vi "GoToKick.vi"(1 "goleiro?":bool, 2 "Impulso ini.\npass state":bool=TRUE, 3 "balls":T4[](array[typedef]), 4 "Robot in in":T5={"id"=0, "function"=enum."Attacker", "x"=0.0, "y"=0.0, "orientation"=0.0, "v_tangent"=0.0, "v_normal"=0.0, "v_ang"=0.0, "kick_x"=0.0, "kick_z"=0.0, "dribble"=FALSE, "Timestamp"=timestamp(0 s since 1904-01-01), "estimatives"={"est_v_tangent"=0.0, "est_v_normal"=0.0, "est_vx"=0.0, "est_vy"=0.0, "Pos Robot Est"=[]}, "dest_x_kick"=0.0, "dest_y_kick"=0.0, "Gap Coord"=[], "States"=enum."Pass", "Path "=[], "Path  Smooth"=[], "Dest"=[]}, 5 "atacando contra?":bool, 6 "Field Size in":T3, 7 "Target":dbl[](array[numeric]), 8 "Defender":bool, 9 "D ball - robot":dbl, 10 "AI Parameters":T2={"GotoKick"={"Dist do cone a frente"=150.0, "attacker farback"=1500.0, "Perto"=300.0, "min dist to kick"=150.0, "kick eps"=0.05, "Time to transition"=0.0}, "Attacker"={"CC chute"=0.09, "CC passe"=0.045, "Kick Force"=100.0, "ball-robot Kick"=200.0, "ball-robot Pass"=0.3, "drible\nAttk"=FALSE}, "Defender"={"D max"=1700.0, "Vel p/ robô av"=1000.0, "Kick Force"=100.0, "D atk-def"=0.0, "D farback"=0.0, "drible\ndef"=FALSE, "drible\ngoalie"=FALSE}, "Timeout"={"Field/v in x"=6.0, "Dist Robots"=300, "Dist up in y"=300}, "Pose Striker"={"dist"=200.0, "Numeric"=-4.0, "dist 2"=200.0, "drible\nstriker"=FALSE}, "Dist Stop"=300.0, "D ball out"=200, "D central gap "=150.0, "T pass"=0.0, "Force ++"=0.0, "range kick"=0.0, "Chute alto"=TRUE, "Marcador novo"=TRUE, "drible"=FALSE, "D drible"=300.0, "Versão Striker"=enum."3", "Defesa"=enum."ManMark", "Marcador"=enum."Marcar Segundo mais perigoso", "Receptor passe"=enum."2nd Striker", "Área"=enum."Quadrada", "Decisão\nsimples?"=FALSE} {"D drible" format="%#_13g"; "D central gap" format="%#_13g"; "Dist Stop" format="%#_13g"; "Pose Striker"."Numeric" format="%#_13g"; "Defender"."Kick Force" format="%#_13g"; "Defender"."Vel p/ robô av" format="%#_13g"; "Attacker"."ball-robot Kick" format="%#_13g"; "Attacker"."Kick Force" format="%#_13g"; "Attacker"."CC passe" format="%#_13g"; "Attacker"."CC chute" format="%#_13g"; "GotoKick"."min dist to kick" format="%#_13g"; "GotoKick"."Perto" format="%#_13g"; "GotoKick"."attacker farback" format="%#_13g"; "GotoKick"."Dist do cone a frente" format="%#_13g"}, 11 "Cone de chute":dbl=0.09 format="%#_13g", 13 "Passe":bool, 16 "Personalidade":T1, 18 "Kick Force":dbl=5.0 format="%#_13g", 19 "IA State Input in":T10) -> (0 "Current States":T7, 12 "Next State":T7, 14 "Robot out":T5={"id"=0, "function"=enum."Attacker", "x"=0.0, "y"=0.0, "orientation"=0.0, "v_tangent"=0.0, "v_normal"=0.0, "v_ang"=0.0, "kick_x"=0.0, "kick_z"=0.0, "dribble"=FALSE, "Timestamp"=timestamp(0 s since 1904-01-01), "estimatives"={"est_v_tangent"=0.0, "est_v_normal"=0.0, "est_vx"=0.0, "est_vy"=0.0, "Pos Robot Est"=[]}, "dest_x_kick"=0.0, "dest_y_kick"=0.0, "Gap Coord"=[], "States"=enum."Pass", "Path "=[], "Path  Smooth"=[], "Dest"=[]}, 17 "kick error":dbl)   [LabVIEW 2018]
uses:
  Core/AI Input.ctl
  Core/AI Robot.ctl
  Functions Enum.ctl
  AttackerStates.ctl
  Path Planning/RRT/PathDests.ctl
  Path Planning/RRT/PathDest.ctl
  Core/AI Ball.ctl
  Core/Field Size.ctl
  Core/AI Judge.ctl
  Command Enum.ctl
  Util/Events/Events.ctl
  AI Parameters.ctl
  PersonalityEnum.ctl
  <vilib>/Analysis/_algsub.llb/Real Vector Norm.vi
  <vilib>/Analysis/baseanly.llb/Real Dot Product.vi
  <vilib>/Analysis/coordinate.llb/2D Cartesian Coordinate Rotation (Scalar).vi
  <vilib>/Analysis/NI_AALPro.lvlib
  <vilib>/Analysis/NI_AALBase.lvlib
panel:
  out "Elapsed Time (s)":dbl
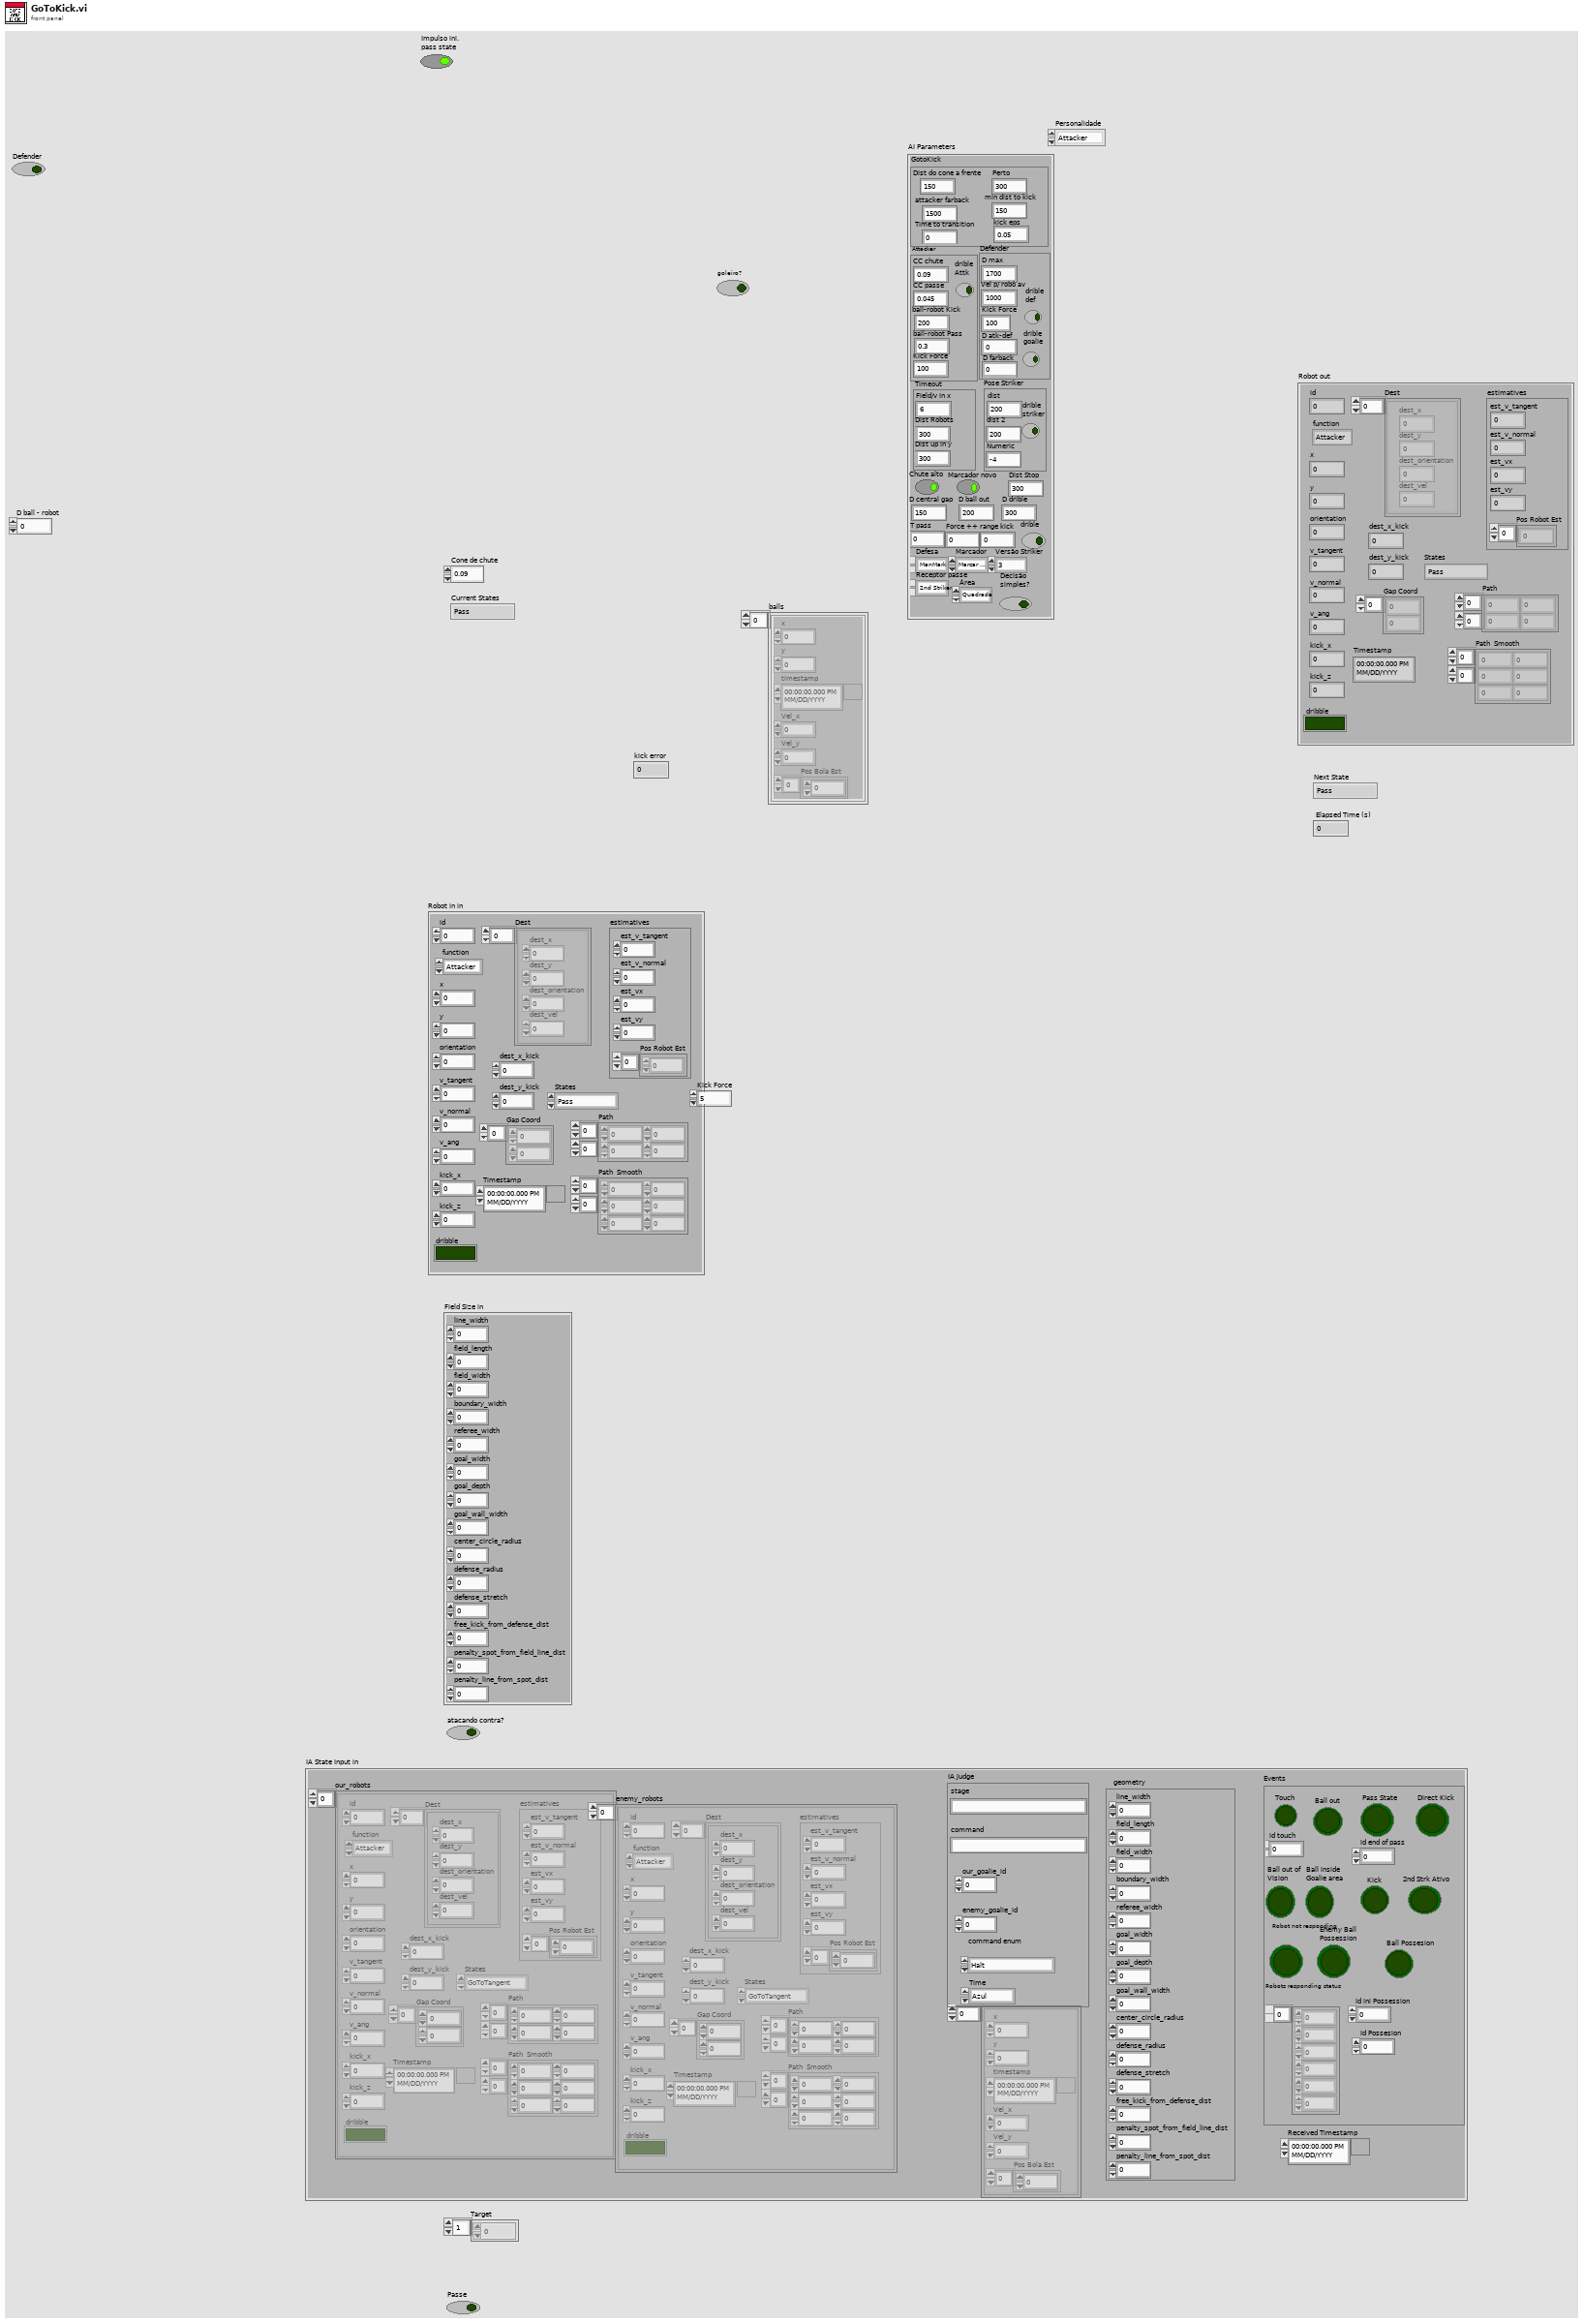
[diagram p1: front panel]
types:
  T1 = typedef "PersonalityEnum.ctl" = enum16{"Attacker", "Striker", "Defender", "Goalie"}
  T2 = typedef "AI Parameters.ctl" = cluster{"GotoKick":cluster{"Dist do cone a frente":dbl, "attacker farback":dbl, "Perto":dbl, "min dist to kick":dbl, "kick eps":dbl, "Time to transition":dbl}, "Attacker":cluster{"CC chute":dbl, "CC passe":dbl, "Kick Force":dbl, "ball-robot Kick":dbl, "ball-robot Pass":dbl, "drible\nAttk":bool}, "Defender":cluster{"D max":dbl, "Vel p/ robô av":dbl, "Kick Force":dbl, "D atk-def":dbl, "D farback":dbl, "drible\ndef":bool, "drible\ngoalie":bool}, "Timeout":cluster{"Field/v in x":dbl, "Dist Robots":u32, "Dist up in y":u32}, "Pose Striker":cluster{"dist":dbl, "Numeric":dbl, "dist 2":dbl, "drible\nstriker":bool}, "Dist Stop":dbl, "D ball out":i32, "D central gap ":dbl, "T pass":dbl, "Force ++":dbl, "range kick":dbl, "Chute alto":bool, "Marcador novo":bool, "drible":bool, "D drible":dbl, "Versão Striker":enum16{"Auto", "3", "2", "1"}, "Defesa":enum16{"ManMark", "Barreira"}, "Marcador":enum16{"Marcar Segundo mais perigoso", "Marcar o mais perigoso"}, "Receptor passe":enum16{"Auto", "2nd Striker", "Striker"}, "Área":enum16{"Quadrada", "Circular"}, "Decisão\nsimples?":bool}
  T3 = typedef "Field Size.ctl" = cluster{"line_width":u32, "field_length":u32, "field_width":u32, "boundary_width":u32, "referee_width":u32, "goal_width":u32, "goal_depth":u32, "goal_wall_width":u32, "center_circle_radius":u32, "defense_radius":u32, "defense_stretch":u32, "free_kick_from_defense_dist":u32, "penalty_spot_from_field_line_dist":u32, "penalty_line_from_spot_dist":u32}
  T4 = typedef "AI Ball.ctl" = cluster{"x":dbl, "y":dbl, "timestamp":timestamp, "Vel_x":dbl, "Vel_y":dbl, "Pos Bola Est":dbl[]}
  T5 = typedef "AI Robot.ctl" = cluster{"id":u32, "function":T6, "x":dbl, "y":dbl, "orientation":dbl, "v_tangent":dbl, "v_normal":dbl, "v_ang":dbl, "kick_x":dbl, "kick_z":dbl, "dribble":bool, "Timestamp":timestamp, "estimatives":cluster{"est_v_tangent":dbl, "est_v_normal":dbl, "est_vx":dbl, "est_vy":dbl, "Pos Robot Est":dbl[]}, "dest_x_kick":dbl, "dest_y_kick":dbl, "Gap Coord":dbl[], "States":T7, "Path ":dbl[][], "Path  Smooth":dbl[][], "Dest":T8}
  T6 = typedef "Functions Enum.ctl" = enum16{"2nd Striker", "Attacker", "Goalie", "Defender", "Striker", "Goto 0", "Dummy", "Kicker", "ZigZag 0", "ZigZag 1", "ZigZag 2", "ZigZag 3", "ZigZag 4", "ZigZag 5", "ZigZag 6", "ZigZag 7", "ZigZag 8", ""}
  T7 = typedef "AttackerStates.ctl" = enum16{"Pass", "GoToTangent", "BallGetting", "GoToKick", ""}
  T8 = typedef "PathDests.ctl" = T9[]
  T9 = typedef "PathDest.ctl" = cluster{"dest_x":dbl, "dest_y":dbl, "dest_orientation":dbl, "dest_vel":dbl}
  T10 = typedef "AI Input.ctl" = cluster{"our_robots":T5[], "enemy_robots":T5[], "balls":T4[], "geometry":T3, "IA Judge":T11, "Received Timestamp":timestamp, "Events":T13}
  T11 = typedef "AI Judge.ctl" = cluster{"stage":string, "command":string, "our_goalie_id":dbl, "enemy_goalie_id":dbl, "command enum":T12, "Time":enum16{"Azul", "Amarelo"}}
  T12 = typedef "Command Enum.ctl" = enum16{"Halt", "Stop", "Force Start", "PKA Normal Start", "Prepare Kickoff Ally", "PKE Normal Start", "Prepare Kickoff Enemy", "Prepare Penalty Ally", "PPA Normal Start", "Prepare Penalty Enemy", "PPE Normal Start", "Direct Free Enemy", "Direct Free Ally", "Indirect Free Enemy", "Indirect Free Ally", "Timeout Enemy", "Timeout Ally", "Goal Enemy", "Goal Ally", "Ball Placement Enemy", "Ball Placement Ally", "Normal Half Time", "Extra Time Break", "Extra Half Time", "None", "Post Game"}
  T13 = typedef "Events.ctl" = cluster{"Touch":bool, "Ball out":bool, "id touch":dbl, "Ball out of \nVision":bool, "Ball inside \nGoalie area":bool, "Robot not responding":bool, "Robots responding status":dbl[], "Enemy Ball \nPossession":bool, "Pass State":bool, "id end of pass":dbl, "Kick":bool, "Id ini Possession":dbl, "Ball Possesion":bool, "Id Possesion":dbl, "Direct Kick":bool, "2nd Strk Ativo":bool}
  T14 = cluster{"Dist do cone a frente":dbl, "attacker farback":dbl, "Perto":dbl, "min dist to kick":dbl, "kick eps":dbl, "Time to transition":dbl}
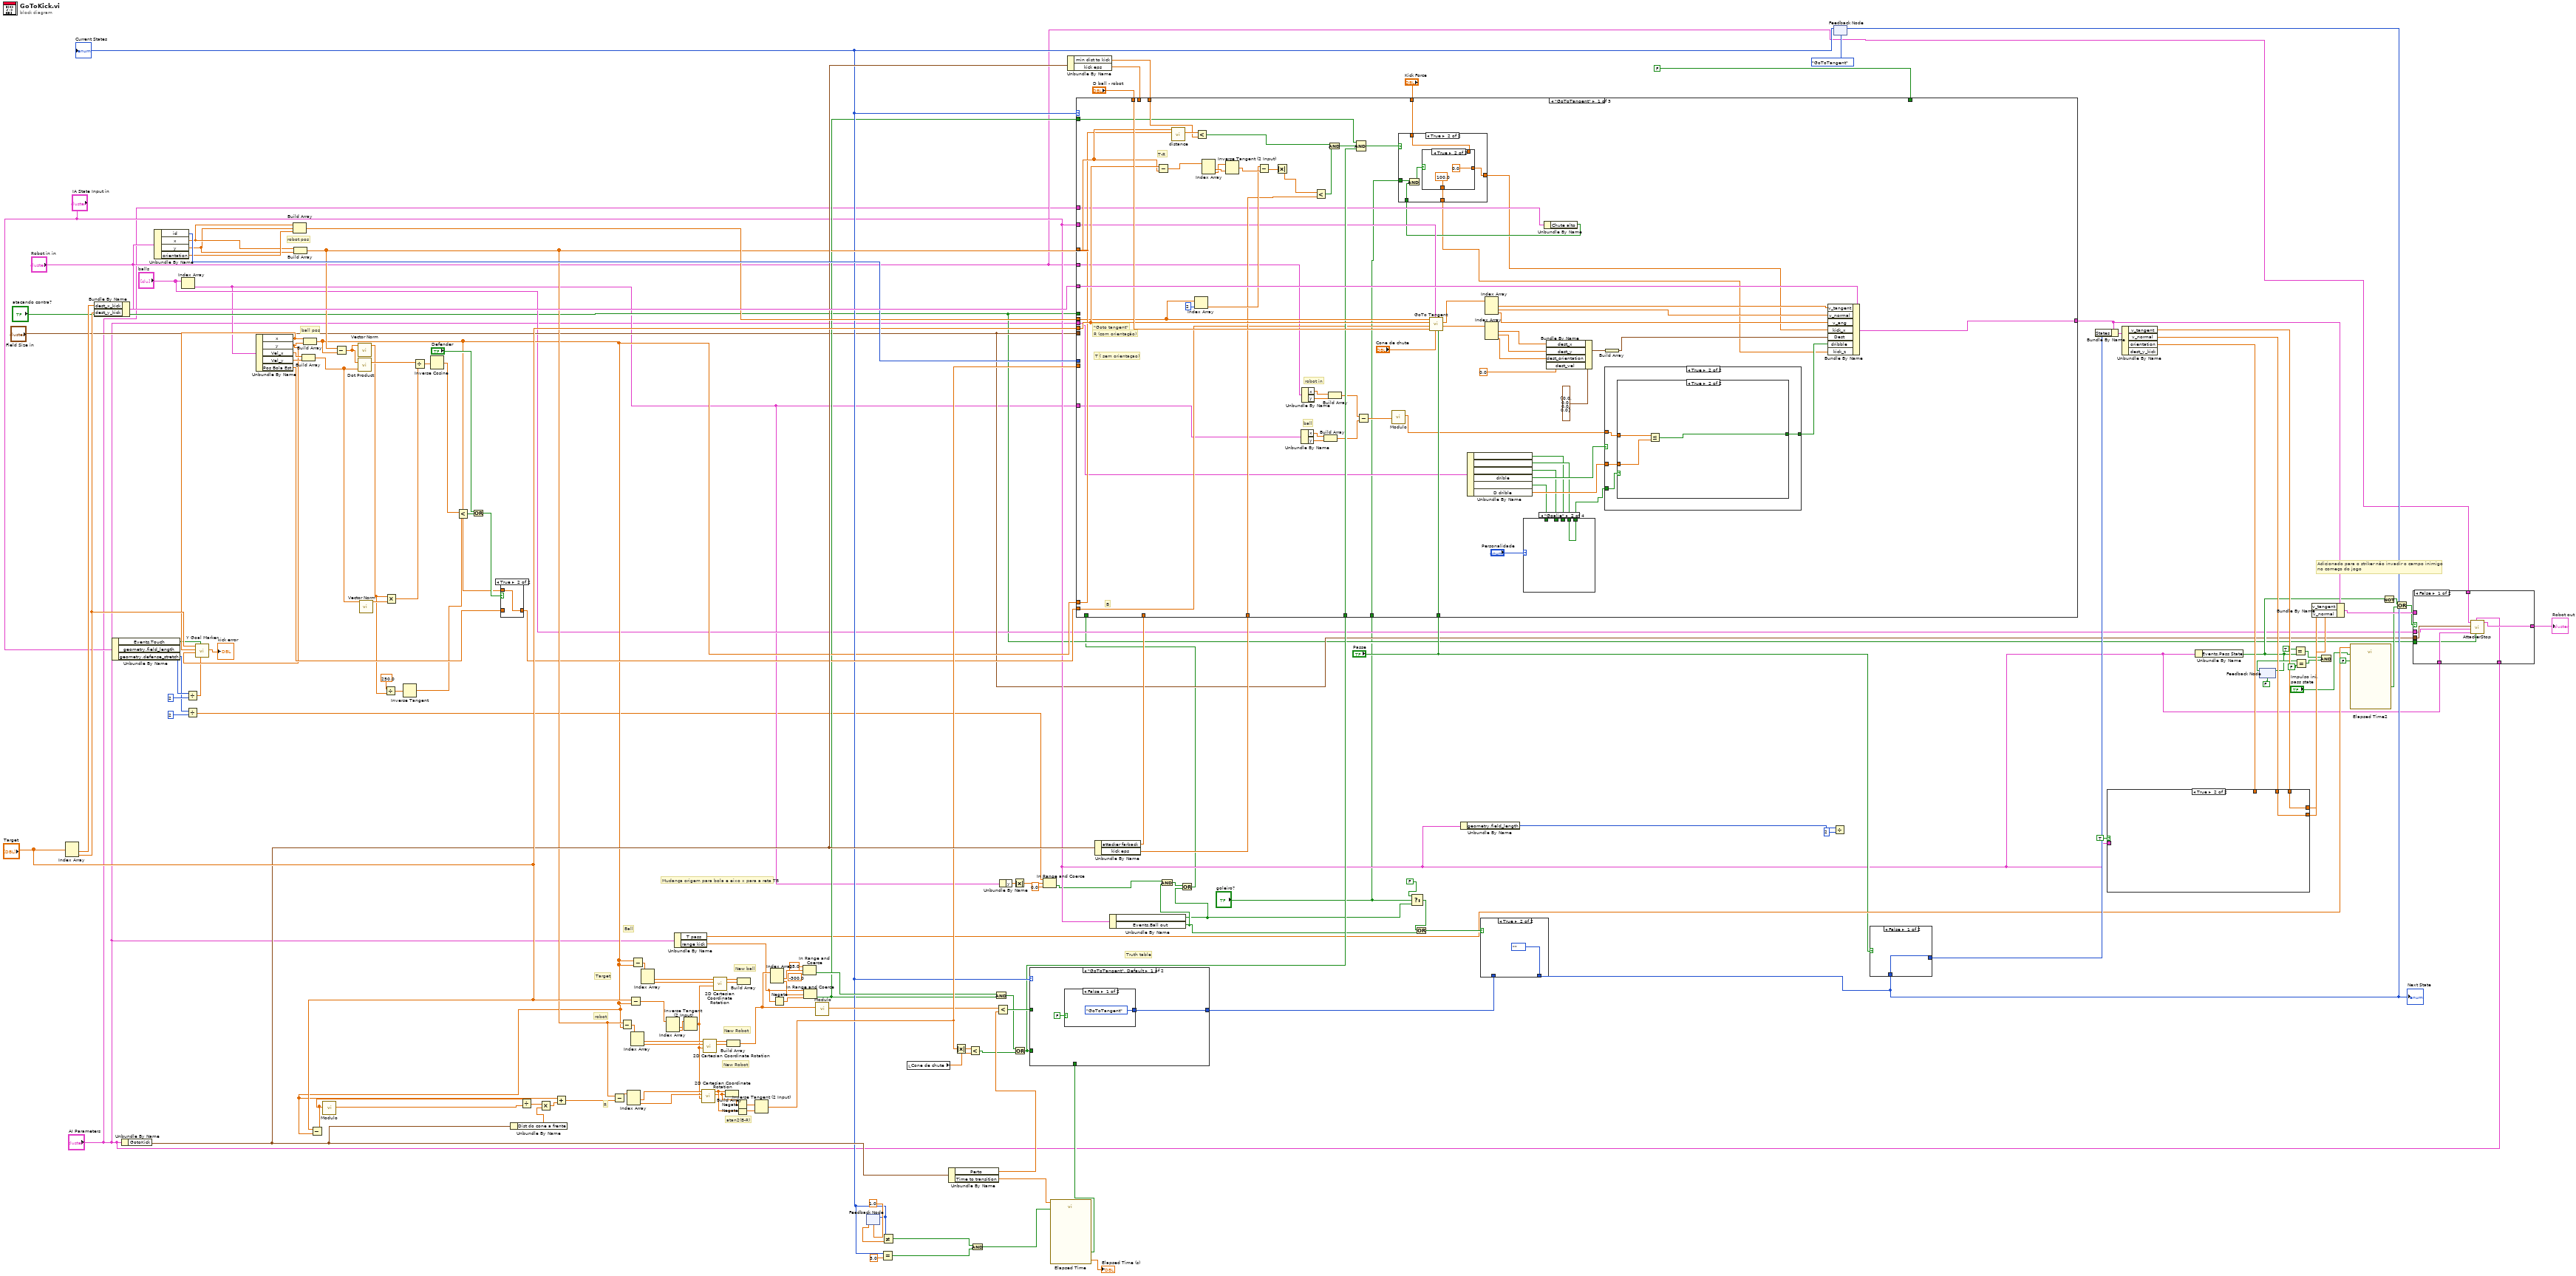
[diagram p0: block diagram]
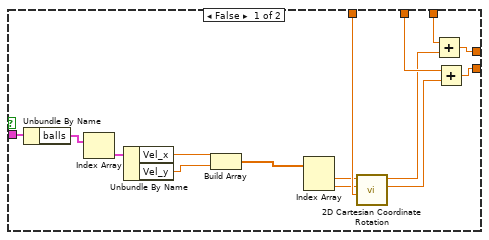
[diagram p3: hidden frame]
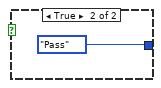
[diagram p5: hidden frame]
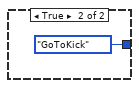
[diagram p6: hidden frame]
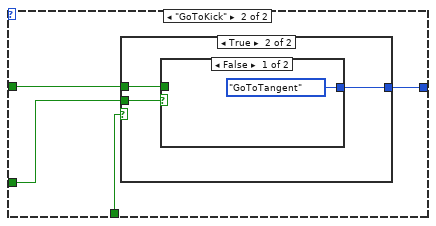
[diagram p7: hidden frame]
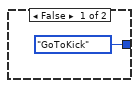
[diagram p8: hidden frame]
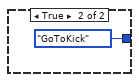
[diagram p9: hidden frame]
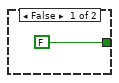
[diagram p14: hidden frame]
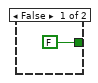
[diagram p15: hidden frame]
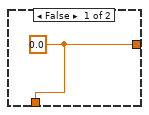
[diagram p16: hidden frame]
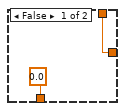
[diagram p17: hidden frame]
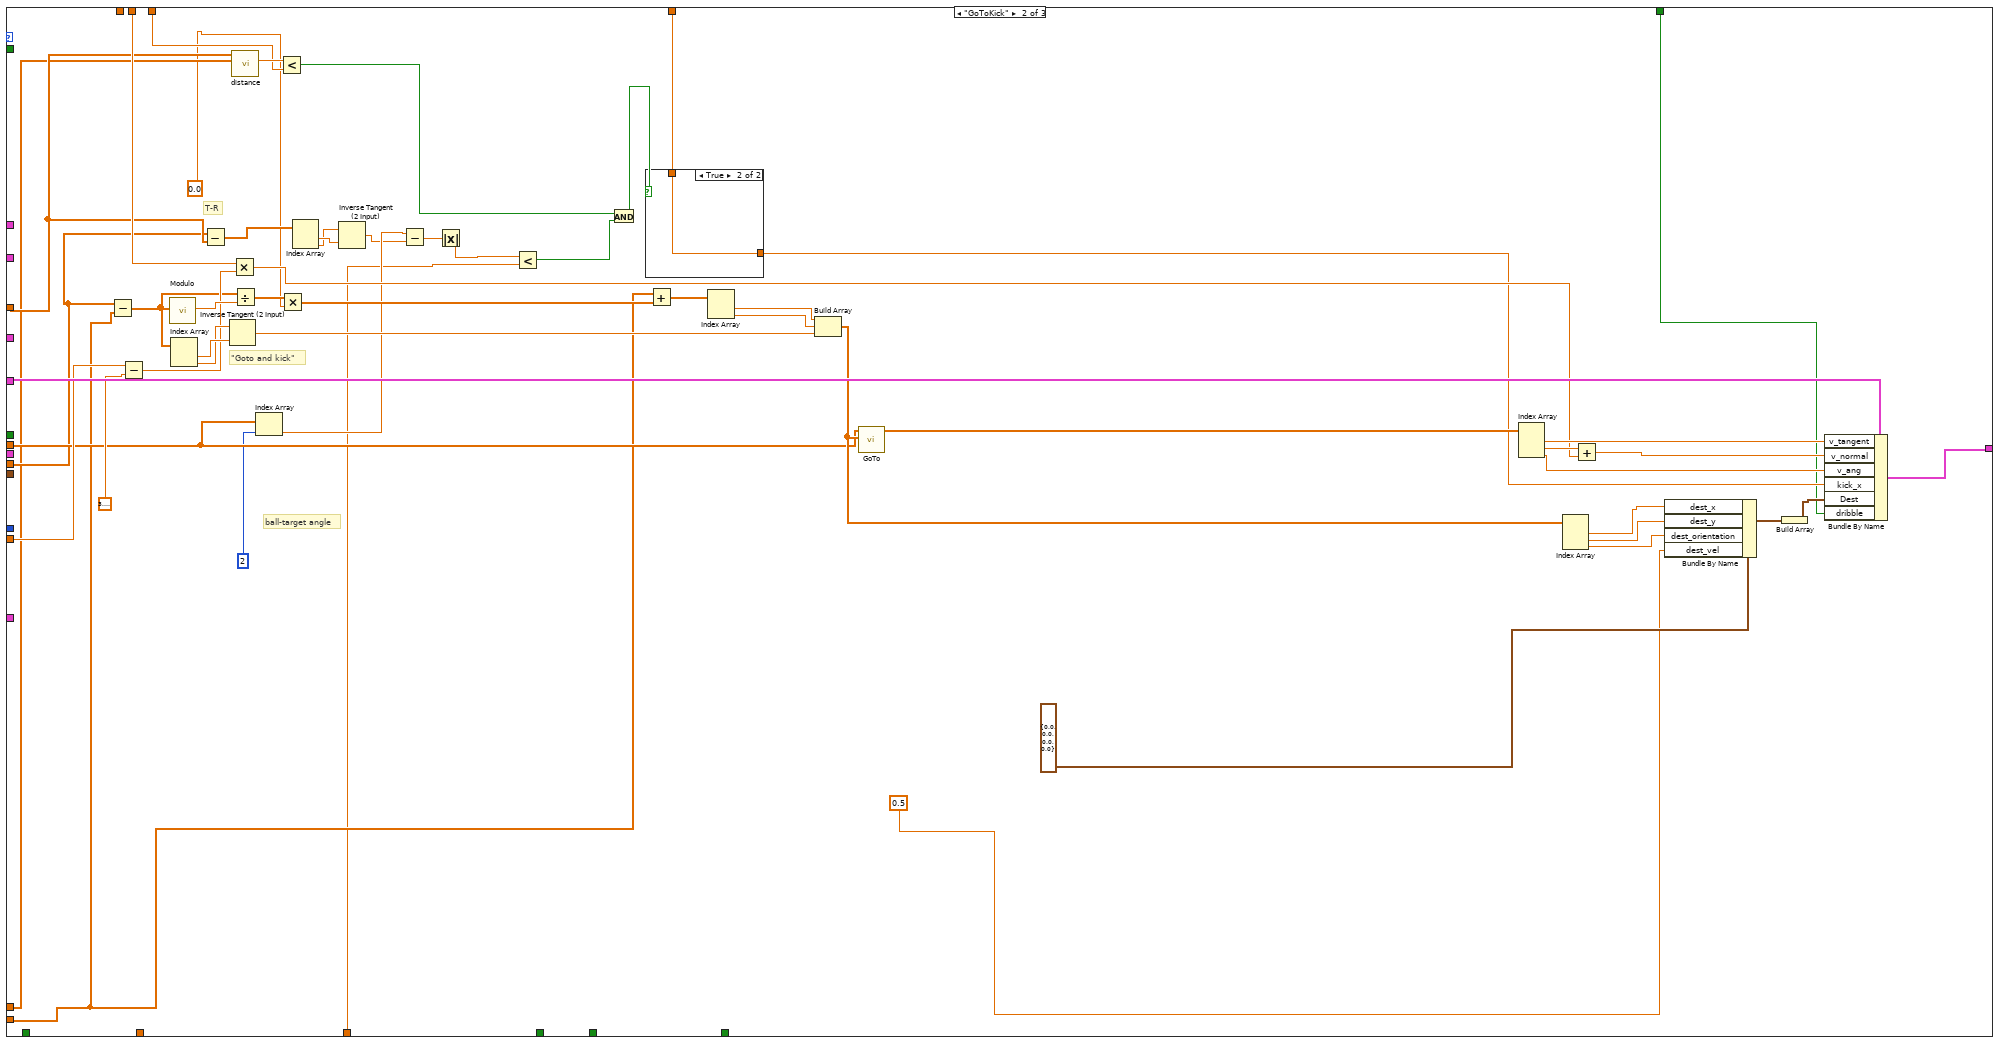
[diagram p18: hidden frame]
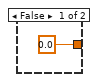
[diagram p19: hidden frame]
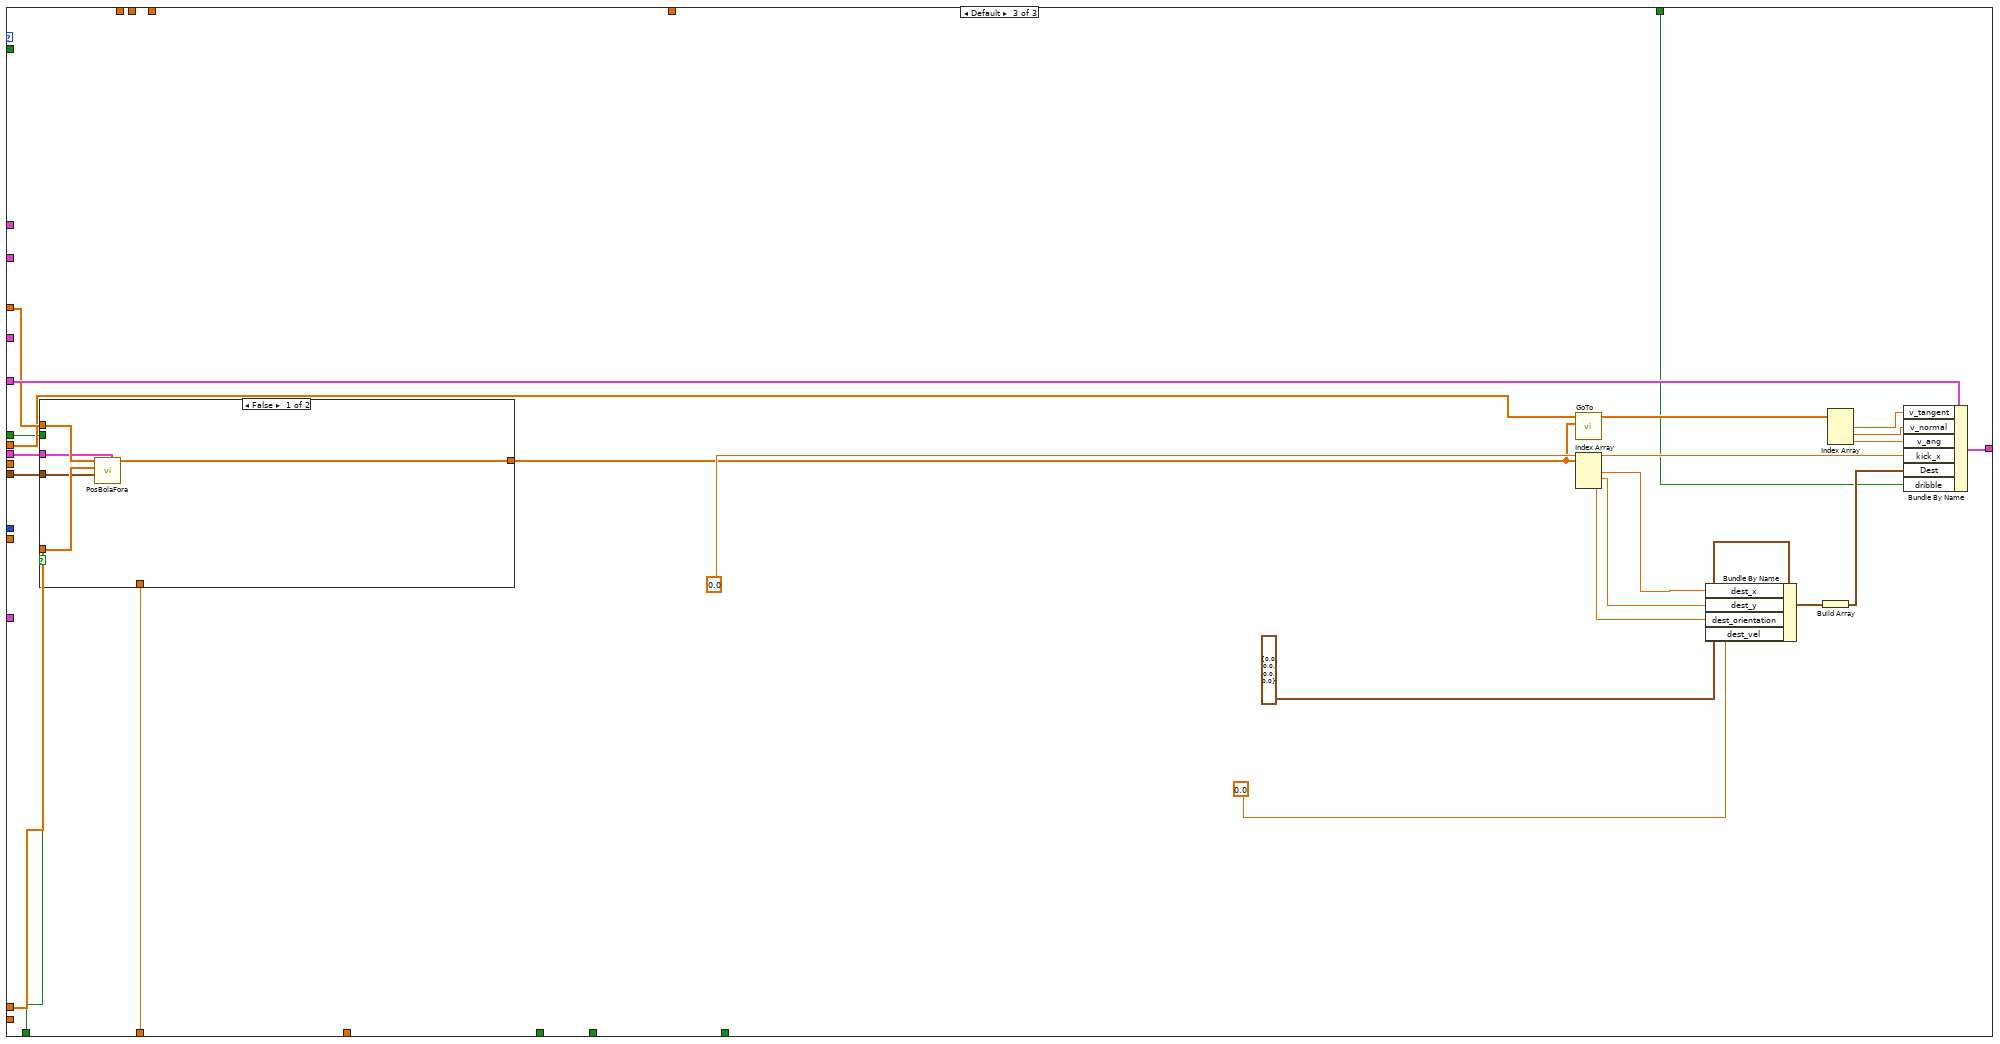
[diagram p20: hidden frame]
diagram:
  # "Adicionado para o striker não invadir o campo inimigo\nno começo do jogo"
  # "New ball"
  # "robot"
  # "atan2(B-R)"
  # "New Robot"
  # "New Robot"
  # "R"
  # "Ball"
  # "Target"
  # "Mudança origem para bola e eixo x para a reta TB"
  # "Truth table"
  # "robot pos"
  # "ball pos"
  n1 = Index Array(array="Target") -> (element #1=w151:dbl, element #2=w54:dbl)  [unwired: 2 in]
  n2 = Bundle By Name(cluster="Robot in in", "dest_x_kick"=w151, "dest_y_kick"=w54) -> (w148:T5)
  n3 = Unbundle By Name("IA State Input in") -> ("Events.Touch"=w51:bool, "geometry.field_length"=w50:u32, "geometry.defense_stretch"=w9:u32)
  n4 = Unbundle By Name("AI Parameters") -> ("GotoKick"=w100:T14)
  n5 = Unbundle By Name("Robot in in") -> ("id"=w126:u32, "x"=w94:dbl, "y"=w93:dbl, "orientation"=w118:dbl)
  n6 = Index Array(array="balls") -> (element=w14:T4)  [unwired: 1 in]
  n7 = Divide(x=w50, y=u32 2) -> (x/y=w48:dbl)
  n8 = Divide(x=w9, y=u32 2) -> (x/y=w8:dbl)
  n9 = Unbundle By Name(w14) -> ("x"=w53:dbl, "y"=w52:dbl, "Vel_x"=w76:dbl, "Vel_y"=w75:dbl, "Pos Bola Est"=w67:dbl[])
  n10 = call "Y Goal Marker.vi"("goal x"=w48, "Touch"=w51, "y"=w52, "x"=w53, "dest_y_kick"=w54) -> ("kick error"=→"kick error":dbl)  [unwired: 6 in]
  n11 = Build Array(w94, w93, w118) -> (w117:dbl[])
  n12 = Build Array(w94, w93) -> (w77:dbl[])
  n13 = Build Array(w76, w75) -> (w73:dbl[])
  n14 = Build Array(w53, w52) -> (w41:dbl[])
  n15 = Subtract(x="Target", y=w41) -> (x-y=w143:dbl[])
  n16 = call "Modulo.vi"("2D vector"=w143) -> ("Modulo"=w142:dbl)  [unwired: 10 in]
  n17 = Subtract(x=w77, y=w41) -> (x-y=w74:dbl[])
  n18 = call-poly <vilib>:"Dot Product.vi"("Y Vector"=w73, "X Vector"=w74) -> ("X * Y"=w70:dbl)  [unwired: 1 out]
  n19 = call-poly <vilib>:"Vector Norm.vi"("Input Vector"=w74) -> ("norm"=w64:dbl)  [unwired: 9 in, 1 out]
  n20 = call-poly <vilib>:"Vector Norm.vi"("Input Vector"=w73) -> ("norm"=w72:dbl)  [unwired: 9 in, 1 out]
  n21 = Divide(x=250.0, y=w64) -> (x/y=w65:dbl)
  n22 = Multiply(x=w64, y=w72) -> (x*y=w71:dbl)
  n23 = Inverse Tangent(1:w65) -> (0:w62:dbl)
  n24 = Divide(x=w70, y=w71) -> (x/y=w69:dbl)
  n25 = Inverse Cosine(1:w69) -> (0:w68:dbl)
  n26 = Less?(x=w68, y=w62) -> (x < y?=w43:bool)
  n27 = Or(x="Defender", y=w43) -> (x .or. y?=w44:bool)
  n28 = case shown="True" w44 {
    tunnel: w67 -> [w152 _]
    tunnel: [w152 w153] -> w66
    tunnel: w41 -> [_ w153]
    frame False {
    }
    frame True {
    }
  }
  n29 = Unbundle By Name(w100) -> ("Dist do cone a frente"=w106:dbl)
  n30 = Divide(x=w143, y=w142) -> (x/y=w141:dbl[])
  n31 = Multiply(x=w141, y=w106) -> (x*y=w140:dbl[])
  n32 = Add(x=w41, y=w140) -> (x+y=w144:dbl[])
  n33 = Subtract(x=w77, y=w144) -> (x-y=w145:dbl[])
  n34 = Subtract(x=w77, y=w41) -> (x-y=w121:dbl[])
  n35 = Index Array(array=w145) -> (element #1=w146:dbl, element #2=w147:dbl)  [unwired: 2 in]
  n36 = Subtract(x="Target", y=w41) -> (x-y=w122:dbl[])
  n37 = Index Array(array=w121) -> (element #1=w119:dbl, element #2=w120:dbl)  [unwired: 2 in]
  n38 = Subtract(x=w41, y=w41) -> (x-y=w90:dbl[])
  n39 = Index Array(array=w90) -> (element #1=w88:dbl, element #2=w89:dbl)  [unwired: 2 in]
  n40 = Index Array(array=w122) -> (element #1=w123:dbl, element #2=w124:dbl)  [unwired: 2 in]
  n41 = Unbundle By Name("AI Parameters") -> ("T pass"=w27:dbl, "range kick"=w28:dbl)
  n42 = Inverse Tangent (2 Input)(1:w123, 2:w124) -> (0:w87:dbl)
  n43 = call-poly <vilib>:"2D Cartesian Coordinate Rotation.vi"("theta"=w87, "y"=w147, "x"=w146) -> ("y out"=w138:dbl, "x out"=w139:dbl)  [unwired: 6 in, 1 out]
  n44 = call-poly <vilib>:"2D Cartesian Coordinate Rotation.vi"("theta"=w87, "y"=w120, "x"=w119) -> ("y out"=w125:dbl, "x out"=w86:dbl)  [unwired: 6 in, 1 out]
  n45 = call-poly <vilib>:"2D Cartesian Coordinate Rotation.vi"("theta"=w87, "y"=w89, "x"=w88) -> ("y out"=w91:dbl, "x out"=w92:dbl)  [unwired: 6 in, 1 out]
  n46 = Build Array(w139, w138) -> ()  [unwired: 1 out]
  n47 = Build Array(w86, w125) -> (w85:dbl[])
  n48 = Negate(x=w138) -> (-x=w136:dbl)
  n49 = Negate(x=w139) -> (-x=w137:dbl)
  n50 = Build Array(w92, w91) -> ()  [unwired: 1 out]
  n51 = Inverse Tangent (2 Input)(1:w137, 2:w136) -> (0:w98:dbl)
  n52 = Index Array(array=w85) -> (element #1=w84:dbl, element #2=w83:dbl)  [unwired: 2 in]
  n53 = Negate(x=w28) -> (-x=w29:dbl)
  n54 = In Range and Coerce(upper limit=25.0, x=w84, lower limit=-300.0) -> (In Range?=w80:bool)  [unwired: 1 out]
  n55 = In Range and Coerce(upper limit=w28, x=w83, lower limit=w29) -> (In Range?=w30:bool)  [unwired: 1 out]
  n56 = call "Modulo.vi"("2D vector"=w85) -> ("Modulo"=w97:dbl)  [unwired: 10 in]
  n57 = feedback #1(1.0 ("Current State")) -> (w132:dbl)
  n58 = local read "Cone de chute"() -> (w46:dbl)
  n59 = Unbundle By Name(w100) -> ("Perto"=w96:dbl, "Time to transition"=w102:dbl)
  n60 = Absolute Value(x=w98) -> (abs(x)=w99:dbl)
  n61 = Less?(x=w99, y=w46) -> (x < y?=w79:bool)
  n62 = And(x=w80, y=w30) -> (x .and. y?=w78:bool)
  n63 = Less?(x=w97, y=w96) -> (x < y?=w95:bool)
  n64 = Unbundle By Name(w14) -> ("y"=w13:dbl)
  n65 = Absolute Value(x=w13) -> (abs(x)=w12:dbl)
  n66 = Or(x=w78, y=w79) -> (x .or. y?=w59:bool)
  n67 = In Range and Coerce(upper limit=w8, x=w12, lower limit=0.0) -> (In Range?=w7:bool)  [unwired: 1 out]
  n68 = Unbundle By Name(w100) -> ("min dist to kick"=w104:dbl, "kick eps"=w103:dbl)
  n69 = Unbundle By Name(w100) -> ("attacker farback"=w105:dbl, "kick eps"=w55:dbl)
  n70 = Unbundle By Name("IA State Input in") -> ("Events.Ball inside \nGoalie area"=w6:bool, "Events.Ball out"=w16:bool)
  n71 = And(x=w7, y=w16) -> (x .and. y?=w15:bool)
  n72 = Or(x=w15, y=w6) -> (x .or. y?=w5:bool)
  n73 = Select(t=FALSE, s="goleiro?", f=w6) -> (s? t:f=w107:bool)
  n74 = Or(x=w107, y=w16) -> (x .or. y?=w135:bool)
  n75 = Unbundle By Name("IA State Input in") -> ("geometry.field_length"=w57:u32)
  n76 = Divide(x=w57, y=u32 2) -> ()  [unwired: 1 out]
  n77 = feedback #2(AttackerStates."GoToTangent" ("Next State")) -> (w61:T7)
  "Current States" <- w61
  n78 = feedback-in #1(w61) -> ()
  n79 = Equal?(x=w61, y=3.0) -> (x = y?=w129:bool)
  n80 = Not Equal?(x=w61, y=w132) -> (x != y?=w130:bool)
  n81 = And(x=w130, y=w129) -> (x .and. y?=w134:bool)
  n82 = call "Elapsed Time"("Time Target (s)"=w102, "Reset"=w134) -> ("Elapsed Time (s)"=→"Elapsed Time (s)":dbl, "Time has Elapsed"=w127:bool)  [unwired: 10 in, 6 out]
  n83 = case shown="\"GoToTangent\", Default" w61 {
    tunnel: [w155 w160] -> w149
    tunnel: w127 -> [_ w161]
    tunnel: w59 -> [_ w159]
    tunnel: w95 -> [_ w158]
    frame "GoToTangent", Default {
      n84 = case shown="False" FALSE {
        tunnel: [AttackerStates."GoToTangent" ("Next State") AttackerStates."GoToKick" ("Next State")] -> w155
        frame False {
        }
        frame True {
        }
      }
    }
    frame "GoToKick" {
      n85 = case shown="True" w161 {
        tunnel: [AttackerStates."GoToKick" ("Next State") w165] -> w160
        tunnel: w159 -> [_ w164]
        tunnel: w158 -> [_ w163]
        frame False {
        }
        frame True {
          n86 = case shown="False" w164 {
            tunnel: [AttackerStates."GoToTangent" ("Next State") AttackerStates."GoToKick" ("Next State")] -> w165
            tunnel: w163 -> [_ _]
            frame False {
            }
            frame True {
            }
          }
        }
      }
    }
  }
  n87 = case shown="\"GoToTangent\"" w61 {
    tunnel: [w227 w310 w336] -> w58
    tunnel: w148 -> [w228 w309 w335]
    tunnel: w117 -> [w210 w279 w329]
    tunnel: w77 -> [w214 w273 w331]
    tunnel: w41 -> [w213 w269 w332]
    tunnel: "Target" -> [w215 w272 _]
    tunnel: "Field Size in" -> [_ _ w330]
    tunnel: w126 -> [_ _ _]
    tunnel: w5 -> [_ _ w326]
    tunnel: "atacando contra?" -> [_ _ w325]
    tunnel: w98 -> [_ w292 _]
    tunnel: w105 -> [_ _ w322]
    tunnel: w104 -> [w212 w287 _]
    tunnel: w103 -> [_ w286 _]
    tunnel: "D ball - robot" -> [w226 _ _]
    tunnel: "AI Parameters" -> [w193 _ w321]
    tunnel: "IA State Input in" -> [w173 _ _]
    tunnel: w66 -> [w203 w270 _]
    tunnel: "Kick Force" -> [w216 w268 _]
    tunnel: w59 -> [w207 _ _]
    tunnel: w55 -> [w205 w267 _]
    tunnel: w30 -> [w202 _ _]
    tunnel: "Passe" -> [w201 _ _]
    tunnel: "Robot in in" -> [w190 _ _]
    tunnel: w14 -> [w189 _ _]
    tunnel: FALSE -> [_ w258 w313]
    tunnel: "goleiro?" -> [w170 _ _]
    tunnel: "AI Parameters" -> [w172 _ _]
    frame "GoToTangent" {
      # "ball"
      # "robot in"
      # "T-R"
      # "\"Goto tangent\""
      # "B"
      # "T"
      # "R ( sem orientaçao)"
      # "R (com orientação)"
      n88 = Subtract(x=w215, y=w214) -> (x-y=w222:dbl[])
      n89 = call "distance.vi"("P1"=w213, "P2"=w214) -> ("Dist P1P2"=w225:dbl)  [unwired: 9 in]
      n90 = Index Array(array=w210, index=2) -> (element=w209:dbl)
      n91 = Less?(x=w225, y=w212) -> (x < y?=w221:bool)
      n92 = Index Array(array=w222) -> (element #1=w224:dbl, element #2=w223:dbl)  [unwired: 2 in]
      n93 = Inverse Tangent (2 Input)(1:w224, 2:w223) -> (0:w220:dbl)
      n94 = Subtract(x=w209, y=w220) -> (x-y=w219:dbl)
      n95 = Absolute Value(x=w219) -> (abs(x)=w217:dbl)
      n96 = Unbundle By Name(w189) -> ("x"=w185:dbl, "y"=w186:dbl)
      n97 = Unbundle By Name(w190) -> ("x"=w188:dbl, "y"=w187:dbl)
      n98 = Less?(x=w217, y=w205) -> (x < y?=w218:bool)
      n99 = Build Array(w185, w186) -> (w183:dbl[])
      n100 = And(x=w221, y=w218) -> (x .and. y?=w208:bool)
      n101 = Build Array(w188, w187) -> (w184:dbl[])
      n102 = Compound Arithmetic op=AND(w202, w208, w207) -> (w206:bool)
      n103 = Subtract(x=w184, y=w183) -> (x-y=w182:dbl[])
      n104 = call "Modulo.vi"("2D vector"=w182) -> ("Modulo"=w181:dbl)  [unwired: 10 in]
      n105 = call "GoTo Tangent.vi"("Passe"=w201, "Cone de chute"="Cone de chute", "IA State Input in"=w173, "distance between ball and robot"=w226, "Ball"=w203, "Target"=w215, "R"=w210) -> ("Destination"=w230:dbl[], "Output\nVelocity"=w231:dbl[])  [unwired: 3 in]
      n106 = Unbundle By Name(w193) -> ("Defender.drible\ndef"=w175:bool, "Defender.drible\ngoalie"=w176:bool, "Pose Striker.drible\nstriker"=w174:bool, "drible"=w192:bool, "Attacker.drible\nAttk"=w177:bool, "D drible"=w180:dbl)
      n107 = Index Array(array=w231) -> (element #1=w233:dbl, element #2=w229:dbl, element #3=w232:dbl)  [unwired: 3 in]
      n108 = Index Array(array=w230) -> (element #1=w196:dbl, element #2=w195:dbl, element #3=w194:dbl)  [unwired: 3 in]
      n109 = case shown="\"Goalie\"" "Personalidade" {
        tunnel: [w234 w235 w236 w237] -> w178
        tunnel: w177 -> [w234 _ _ _]
        tunnel: w176 -> [_ w235 _ _]
        tunnel: w175 -> [_ _ w236 _]
        tunnel: w174 -> [_ _ _ w237]
        frame "Attacker", Default {
        }
        frame "Goalie" {
        }
        frame "Defender" {
        }
        frame "Striker" {
        }
      }
      n110 = Unbundle By Name(w172) -> ("Chute alto"=w171:bool)
      n111 = case shown="True" w206 {
        tunnel: [w247 w250] -> w169
        tunnel: w216 -> [_ w248]
        tunnel: w171 -> [_ w253]
        tunnel: w170 -> [_ w252]
        tunnel: [w247 w249] -> w168
        frame False {
          w247 = 0.0
        }
        frame True {
          n112 = And(x=w252, y=w253) -> (x .and. y?=w251:bool)
          n113 = case shown="True" w251 {
            tunnel: [w254 0.0] -> w250
            tunnel: [0.0 100.0] -> w249
            tunnel: w248 -> [w254 _]
            frame False {
            }
            frame True {
            }
          }
        }
      }
      n114 = Bundle By Name(cluster=T9 {"dest_x"=0.0, "dest_y"=0.0, "dest_orientation"=0.0, "dest_vel"=0.0} ("Dest"), "dest_x"=w196, "dest_y"=w195, "dest_orientation"=w194, "dest_vel"=0.0) -> (w199:T9)
      n115 = case shown="True" w192 {
        tunnel: [FALSE w241] -> w191
        tunnel: w178 -> [_ w242]
        tunnel: w181 -> [_ w240]
        tunnel: w180 -> [_ w239]
        frame False {
        }
        frame True {
          n116 = case shown="True" w242 {
            tunnel: [FALSE w244] -> w241
            tunnel: w240 -> [_ w246]
            tunnel: w239 -> [_ w245]
            frame False {
            }
            frame True {
              n117 = Less Or Equal?(x=w246, y=w245) -> (x <= y?=w244:bool)
            }
          }
        }
      }
      n118 = Build Array(w199) -> (w197:T9[])
      n119 = Bundle By Name(cluster=w228, "v_tangent"=w233, "v_normal"=w229, "v_ang"=w232, "kick_x"=w169, "Dest"=w197, "dribble"=w191, "kick_z"=w168) -> (w227:T5)
    }
    frame "GoToKick" {
      # "T-R"
      # "ball-target angle"
      # "\"Goto and kick\""
      n120 = Subtract(x=w272, y=w270) -> (x-y=w283:dbl[])
      n121 = Subtract(x=w292, y=3.141592653589793) -> (x-y=w290:dbl)
      n122 = call "Modulo.vi"("2D vector"=w283) -> ("Modulo"=w297:dbl)  [unwired: 10 in]
      n123 = Index Array(array=w283) -> (element #1=w307:dbl, element #2=w306:dbl)  [unwired: 2 in]
      n124 = Subtract(x=w272, y=w273) -> (x-y=w282:dbl[])
      n125 = Inverse Tangent (2 Input)(1:w307, 2:w306) -> (0:w305:dbl)
      n126 = Multiply(x=w286, y=w290) -> (x*y=w293:dbl)
      n127 = call "distance.vi"("P1"=w269, "P2"=w273) -> ("Dist P1P2"=w308:dbl)  [unwired: 9 in]
      n128 = Divide(x=w283, y=w297) -> (x/y=w298:dbl[])
      n129 = Index Array(array=w279, index=2) -> (element=w277:dbl)
      n130 = Less?(x=w308, y=w287) -> (x < y?=w281:bool)
      n131 = Multiply(x=w298, y=0.0) -> (x*y=w300:dbl[])
      n132 = Index Array(array=w282) -> (element #1=w285:dbl, element #2=w284:dbl)  [unwired: 2 in]
      n133 = Inverse Tangent (2 Input)(1:w285, 2:w284) -> (0:w276:dbl)
      n134 = Subtract(x=w277, y=w276) -> (x-y=w275:dbl)
      n135 = Absolute Value(x=w275) -> (abs(x)=w271:dbl)
      n136 = Less?(x=w271, y=w267) -> (x < y?=w274:bool)
      n137 = And(x=w281, y=w274) -> (x .and. y?=w280:bool)
      n138 = case shown="True" w280 {
        tunnel: [0.0 w312] -> w289
        tunnel: w268 -> [_ w312]
        frame False {
        }
        frame True {
        }
      }
      n139 = Add(x=w270, y=w300) -> (x+y=w299:dbl[])
      n140 = Index Array(array=w299) -> (element #1=w304:dbl, element #2=w303:dbl)  [unwired: 2 in]
      n141 = Build Array(w304, w303, w305) -> (w296:dbl[])
      n142 = call "GoTo.vi"("Target"=w296, "Position"=w279) -> ("Output\nVelocity"=w302:dbl[])  [unwired: 8 in, 1 out]
      n143 = Index Array(array=w302) -> (element #1=w301:dbl, element #2=w295:dbl, element #3=w288:dbl)  [unwired: 3 in]
      n144 = Index Array(array=w296) -> (element #1=w262:dbl, element #2=w261:dbl, element #3=w260:dbl)  [unwired: 3 in]
      n145 = Add(x=w295, y=w293) -> (x+y=w294:dbl)
      n146 = Bundle By Name(cluster=T9 {"dest_x"=0.0, "dest_y"=0.0, "dest_orientation"=0.0, "dest_vel"=0.0} ("Dest"), "dest_x"=w262, "dest_y"=w261, "dest_orientation"=w260, "dest_vel"=0.5) -> (w264:T9)
      n147 = Build Array(w264) -> (w263:T9[])
      n148 = Bundle By Name(cluster=w309, "v_tangent"=w301, "v_normal"=w294, "v_ang"=w288, "kick_x"=w289, "Dest"=w263, "dribble"=w258) -> (w310:T5)
    }
    frame Default {
      n149 = case shown="False" w326 {
        tunnel: w332 -> [w341 w352]
        tunnel: w331 -> [w340 w350]
        tunnel: w330 -> [w339 w351]
        tunnel: [w338 w357] -> w327
        tunnel: w325 -> [_ _]
        tunnel: w322 -> [_ w343]
        tunnel: w321 -> [w337 _]
        frame False {
          n150 = call "PosBolaFora.vi"("AI Parameters"=w337, "Field Size in"=w339, "Position da bola"=w341, "Position do robot"=w340) -> ("Target"=w338:dbl[])  [unwired: 7 in]
        }
        frame True {
          # "ball-target angle"
          n151 = Unbundle By Name(w351) -> ("field_length"=w349:u32)
          n152 = Subtract(x=w352, y=w350) -> (x-y=w355:dbl[])
          n153 = Index Array(array=w352) -> (element #1=w346:dbl, element #2=w358:dbl)  [unwired: 2 in]
          n154 = Index Array(array=w355) -> (element #1=w353:dbl, element #2=w354:dbl)  [unwired: 2 in]
          n155 = Divide(x=w349, y=u32 2) -> (x/y=w347:dbl)
          n156 = Inverse Tangent (2 Input)(1:w353, 2:w354) -> (0:w342:dbl)
          n157 = Subtract(x=w347, y=w343) -> (x-y=w345:dbl)
          n158 = Sign(1:w346) -> (0:w344:dbl)
          n159 = Multiply(x=w345, y=w344) -> (x*y=w356:dbl)
          n160 = Build Array(w356, w358, w342) -> (w357:dbl[])
        }
      }
      n161 = call "GoTo.vi"("Target"=w327, "Position"=w329) -> ("Output\nVelocity"=w328:dbl[])  [unwired: 8 in, 1 out]
      n162 = Index Array(array=w327) -> (element #1=w316:dbl, element #2=w315:dbl, element #3=w314:dbl)  [unwired: 3 in]
      n163 = Bundle By Name(cluster=T9 {"dest_x"=0.0, "dest_y"=0.0, "dest_orientation"=0.0, "dest_vel"=0.0} ("Dest"), "dest_x"=w316, "dest_y"=w315, "dest_orientation"=w314, "dest_vel"=0.0) -> (w319:T9)
      n164 = Build Array(w319) -> (w317:T9[])
      n165 = Index Array(array=w328) -> (element #1=w333:dbl, element #2=w324:dbl, element #3=w323:dbl)  [unwired: 3 in]
      n166 = Bundle By Name(cluster=w335, "v_tangent"=w333, "v_normal"=w324, "v_ang"=w323, "kick_x"=0.0, "Dest"=w317, "dribble"=w313) -> (w336:T5)
    }
  }
  n167 = case shown="True" w135 {
    tunnel: [w359 AttackerStates."" ("Next State")] -> w116
    tunnel: w149 -> [w359 _]
    frame False {
    }
    frame True {
    }
  }
  "Next State" <- w116
  n168 = feedback-in #2(w116) -> ()
  n169 = case shown="False" "Passe" {
    tunnel: w116 -> [w361 _]
    tunnel: [w361 AttackerStates."Pass" ("Next State")] -> w150
    frame False {
    }
    frame True {
    }
  }
  n170 = Bundle By Name(cluster=w58, "States"=w150) -> (w114:T5)
  n171 = Unbundle By Name(w114) -> ("v_tangent"=w112:dbl, "v_normal"=w111:dbl, "orientation"=w113:dbl)  [unwired: 1 out]
  n172 = case shown="True" TRUE {
    tunnel: w113 -> [w377 _]
    tunnel: w112 -> [w376 w379]
    tunnel: w111 -> [w375 w378]
    tunnel: [w374 w378] -> w110
    tunnel: [w373 w379] -> w109
    tunnel: "IA State Input in" -> [w372 _]
    frame False {
      n173 = Unbundle By Name(w372) -> ("balls"=w371:T4[])
      n174 = Index Array(array=w371) -> (element=w370:T4)  [unwired: 1 in]
      n175 = Unbundle By Name(w370) -> ("Vel_x"=w366:dbl, "Vel_y"=w365:dbl)
      n176 = Build Array(w366, w365) -> (w367:dbl[])
      n177 = Index Array(array=w367) -> (element #1=w369:dbl, element #2=w368:dbl)  [unwired: 2 in]
      n178 = call-poly <vilib>:"2D Cartesian Coordinate Rotation.vi"("theta"=w377, "y"=w368, "x"=w369) -> ("y out"=w363:dbl, "x out"=w364:dbl)  [unwired: 6 in, 1 out]
      n179 = Add(x=w376, y=w364) -> (x+y=w373:dbl)
      n180 = Add(x=w375, y=w363) -> (x+y=w374:dbl)
    }
    frame True {
    }
  }
  n181 = Unbundle By Name("IA State Input in") -> ("Events.Pass State"=w24:bool)
  n182 = feedback-in #3(w24) -> ()
  n183 = feedback #3(FALSE ("Pass State")) -> (w35:bool)
  n184 = Equal?(x=TRUE, y=w24) -> (x = y?=w32:bool)
  n185 = Equal?(x=w35, y=FALSE) -> (x = y?=w31:bool)
  n186 = Bundle By Name(cluster=w58, "v_tangent"=w109, "v_normal"=w110) -> (w39:T5)
  n187 = And(x=w32, y=w31) -> ()  [unwired: 1 out]
  n188 = call "Elapsed Time2"("Time Target (s)"=w27, "Reset"="Impulso ini.\npass state", "Auto Reset"=FALSE) -> ("Time has Elapsed"=w23:bool)  [unwired: 9 in, 7 out]
  n189 = Not(x=w24) -> (.not. x?=w25:bool)
  n190 = Or(x=w25, y=w23) -> (x .or. y?=w22:bool)
  n191 = case shown="False" w22 {
    tunnel: w39 -> [_ w387]
    tunnel: [w384 w387] -> w38
    tunnel: "IA State Input in" -> [w386 _]
    tunnel: "Robot in in" -> [w385 _]
    tunnel: "Field Size in" -> [w383 _]
    tunnel: "balls" -> [w382 _]
    tunnel: "AI Parameters" -> [w381 _]
    tunnel: "atacando contra?" -> [w380 _]
    frame False {
      n192 = call "AttackerStop.vi"("atacando contra?"=w380, "AI Parameters"=w381, "IA State Input 2"=w386, "balls"=w382, "Field Size in"=w383, "Robot in"=w385) -> ("Robot out"=w384:T5)  [unwired: 5 in]
    }
    frame True {
    }
  }
  "Robot out" <- w38
